vi "DevB.Off.vi"(8 "error in (no error)":errorcluster, 10 "off":bool=TRUE, 11 "DevB Session in":T1) -> (0 "error out":errorcluster, 3 "DevB Session out":T1)   [LabVIEW 2018]
uses:
  typedefs/DevB.Session.ctl
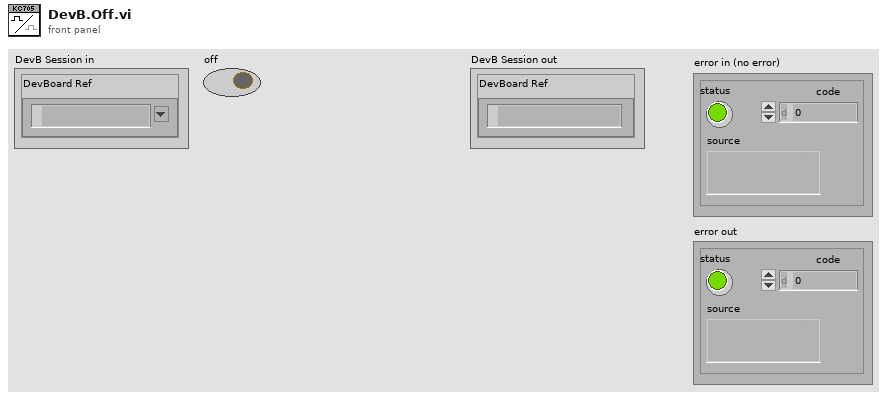
[diagram p1: front panel]
types:
  T1 = typedef "DevB.Session.ctl" = cluster{"DevBoard Ref":refnum<visa-resource-name>}
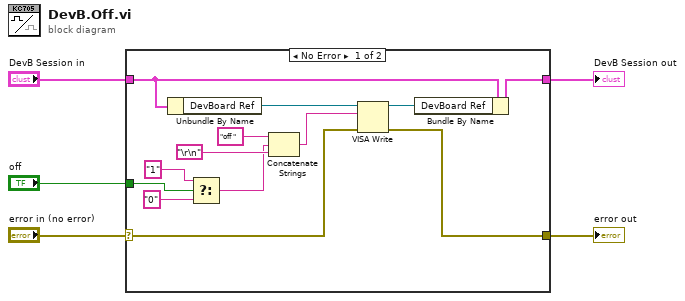
[diagram p0: block diagram]
diagram:
  n1 = case shown="No Error" "error in (no error)" {
    selector: "error in (no error)" -> [w15 w20]
    tunnel: "DevB Session in" -> [w17 w19]
    tunnel: [w14 w20] -> w3
    tunnel: [w13 w19] -> w2
    tunnel: "off" -> [w9 _]
    frame No Error {
      n2 = Unbundle By Name(w17) -> ("DevBoard Ref"=w18:refnum<visa-resource-name>)
      n3 = Select(t="1", s=w9, f="0") -> (s? t:f=w6:string)
      n4 = Concatenate Strings("off ", w6, "\r\n") -> (w11:string)
      n5 = VISA Write(VISA resource name=w18, write buffer=w11, error in (no error)=w15) -> (VISA resource name out=w16:refnum<visa-resource-name>, error out=w14:errorcluster)  [unwired: 1 out]
      n6 = Bundle By Name(cluster=w17, "DevBoard Ref"=w16) -> (w13:T1)
    }
    frame Error {
    }
  }
  "DevB Session out" <- w2
  "error out" <- w3
